vi "Roller Latch.vi"(1 "Make False":bool, 2 "Make True":bool) -> (0 "Output":bool)   [LabVIEW 2013]
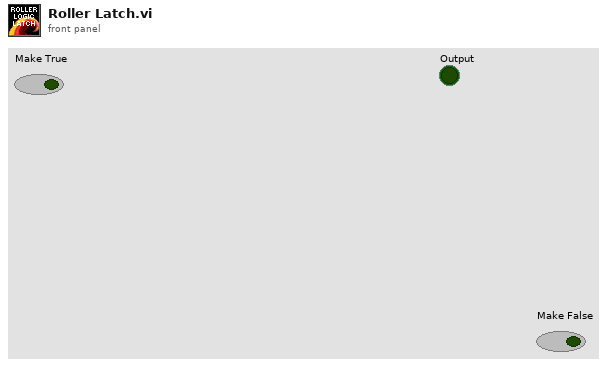
[diagram p1: front panel]
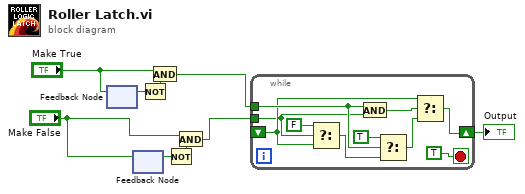
[diagram p0: block diagram]
diagram:
  n1 = feedback-in #1("Make True") -> ()
  n2 = feedback #1() -> (w7:bool)  [unwired: 1 in]
  n3 = feedback #2() -> (w3:bool)  [unwired: 1 in]
  n4 = feedback-in #2("Make False") -> ()
  n5 = Not(x=w7) -> (.not. x?=w6:bool)
  n6 = And(x="Make True", y=w6) -> (x .and. y?=w5:bool)
  n7 = Not(x=w3) -> (.not. x?=w4:bool)
  n8 = And(x="Make False", y=w4) -> (x .and. y?=w2:bool)
  n9 = while {
    tunnel: w2 -> [w10]
    tunnel: w5 -> [w16]
    shift-right: [w17] -> w9
    shift-left: _ -> [w11]
    stop <- TRUE stop-if-true
    n10 = Select(t=FALSE, s=w10, f=w11) -> (s? t:f=w12:bool)
    n11 = And(x=w16, y=w10) -> (x .and. y?=w18:bool)
    n12 = Select(t=TRUE, s=w16, f=w12) -> (s? t:f=w13:bool)
    n13 = Select(t=w11, s=w18, f=w13) -> (s? t:f=w17:bool)
  }
  "Output" <- w9
